vi "Write Log Line.vi"(10 "log line":string, 11 "handler in":refnum<class "Handler.lvclass">) -> (0 "error out":errorcluster, 3 "handler out":refnum<class "Handler.lvclass">)   [LabVIEW 2024, in "Logging.lvlib" / "Handler.lvclass"]
uses:
  Handler.lvclass
  Handler.lvclass/Handler.ctl
  <vilib>/ErrorRing/Error Ring.xnode
panel:
  # "Connector Pane"
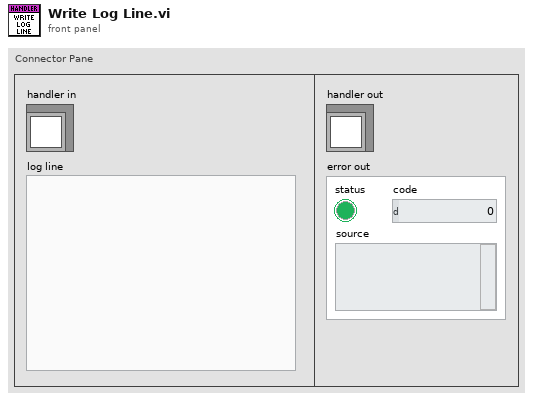
[diagram p1: front panel]
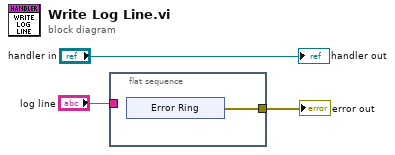
[diagram p0: block diagram]
diagram:
  n1 = flat-sequence {
    tunnel: "log line" -> [_]
    tunnel: [w4] -> w1
    frame #0 {
      n2 = xnode "Error Ring"() -> ("error out"=w4:errorcluster)
    }
  }
  "handler out" <- "handler in"
  "error out" <- w1
